vi "Check Object Lengths.vi"(8 "error in (no error)":errorcluster, 11 "objects in":cluster{"object ID":u8, "value":string}[](array[cluster]) {"object ID" format="%x"}) -> (0 "error out":errorcluster, 3 "objects out":cluster{"object ID":u8, "value":string}[](array[cluster]) {"object ID" format="%x"})   [LabVIEW 2017, in "SubVIs.lvlib" / "Device Data Model.lvclass"]
doc: "Checks to ensure that all Modbus objects can fit within the length allowed by the Modbus protocol data unit and will throw an error if any object is longer than allowed. This check must be performed because objects may not be split across multiple data units, although a request for multiple objects can be split across multiple responses."
uses:
  <vilib>/Modbus/subvis/Data and Functions/Device Data Model/Device Data Model.lvclass
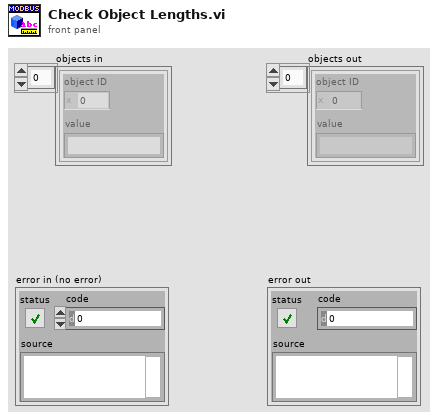
[diagram p1: front panel]
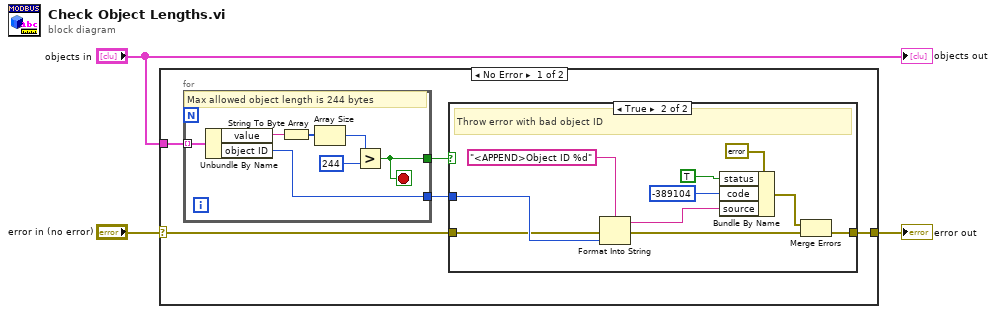
[diagram p0: block diagram]
diagram:
  n1 = case shown="No Error" "error in (no error)" {
    selector: "error in (no error)" -> [w6 w27]
    tunnel: [w5 w27] -> w2
    tunnel: "objects in" -> [w8 _]
    frame No Error {
      n2 = for {
        tunnel: w8 -> [w26] mode=indexing
        tunnel: [w21] -> w7
        tunnel: [w20] -> w4
        stop <- w21 stop-if-true
        # "Max allowed object length is 244 bytes"
        n3 = Unbundle By Name(w26) -> ("value"=w25:string, "object ID"=w20:u8)
        n4 = String To Byte Array(string=w25) -> (unsigned byte array=w24:u8[])
        n5 = Array Size(array=w24) -> (size(s)=w23:i32)
        n6 = Greater?(x=w23, y=244) -> (0:w21:bool)
      }
      n7 = case shown="True" w7 {
        tunnel: w6 -> [w9 w12]
        tunnel: [w9 w17] -> w5
        tunnel: w4 -> [_ w19]
        frame False {
        }
        frame True {
          # "Throw error with bad object ID"
          n8 = Format Into String(format string="<APPEND>Object ID %d", error in=w12, w19) -> (resulting string=w14:string, error out=w11:errorcluster)  [unwired: 1 in]
          n9 = Bundle By Name(cluster=errorcluster {"status"=FALSE, "code"=0, "source"=""} ("error constant"), "status"=TRUE, "code"=-389104 ("error code (0)"), "source"=w14) -> (w10:errorcluster)
          n10 = Merge Errors(w10, w11) -> (w17:errorcluster)
        }
      }
    }
    frame Error {
    }
  }
  "error out" <- w2
  "objects out" <- "objects in"
